vi "Shoot High Goal State Machine.vi"   [LabVIEW 2013]
uses:
  typedefs/DevRef Type.ctl
  typedefs/fg_typedef.ctl
  typedefs/State Machine/subStates.ctl
  typedefs/State Machine/singleUseSubstate.ctl
  <vilib>/Rock Robotics/WPI/Solenoid/WPI_SolenoidValue.ctl
  <vilib>/Rock Robotics/WPI/Solenoid/WPI_SolenoidGetEnum.vi
panel:
  # "A State Machine to Handle a High Goal Shot"
types:
  T1 = typedef "fg_typedef.ctl" = enum16{"Get", "Set"}
  T2 = typedef "DevRef Type.ctl" = enum16{"Shooter Solenoid", "Latch Solenoid", "Right Up Sensor", "Right Down Sensor", "Hold Sensor", "Arm Encoder"}
  T3 = typedef "subStates.ctl" = enum16{"null", "wait", "driver control", "auto", "manual override", "hold position", "rotate", "pickup", "pass", "recover pass", "load", "goto shoot", "shoot high goal", "shoot low goal", "cancel arm", "cancel shooter", "end", "test"}
  T4 = typedef "WPI_SolenoidValue.ctl" = enum16{"Off", "On", "Forward", "Reverse"}
  T5 = typedef "singleUseSubstate.ctl" = enum16{"null", "wait", "shift high", "shift low", "extend shooter", "retract shooter", "latch", "unlatch", "end"}
  T6 = typedef "WPI_DigitalInputDevRef.ctl" = cluster{"DevStatus":errorcluster, "DIO Channel":T7, "Digital Module":T8}
  T7 = typedef "FPGA_DIOChannel.ctl" = enum8{"DIO 1", "DIO 2", "DIO 3", "DIO 4", "DIO 5", "DIO 6", "DIO 7", "DIO 8", "DIO 9", "DIO 10", "DIO 11", "DIO 12", "DIO 13", "DIO 14", "Invalid"}
  T8 = typedef "FPGA_TypedefDigitalModule.ctl" = enum16{"Digital Module 1", "Digital Module 2"}
  T9 = typedef "WPI_SolenoidDevRef.ctl" = cluster{"DevStatus":errorcluster, "Solenoid Module":T10, "Forward Solenoid Channel":T11, "Reverse Solenoid Channel":T11}
  T10 = typedef "FPGA_TypedefSolenoidModule.ctl" = enum16{"Solenoid Module 1", "Solenoid Module 2"}
  T11 = typedef "WPI_SolenoidChannel.ctl" = enum8{"Solenoid 1", "Solenoid 2", "Solenoid 3", "Solenoid 4", "Solenoid 5", "Solenoid 6", "Solenoid 7", "Solenoid 8", "Invalid"}
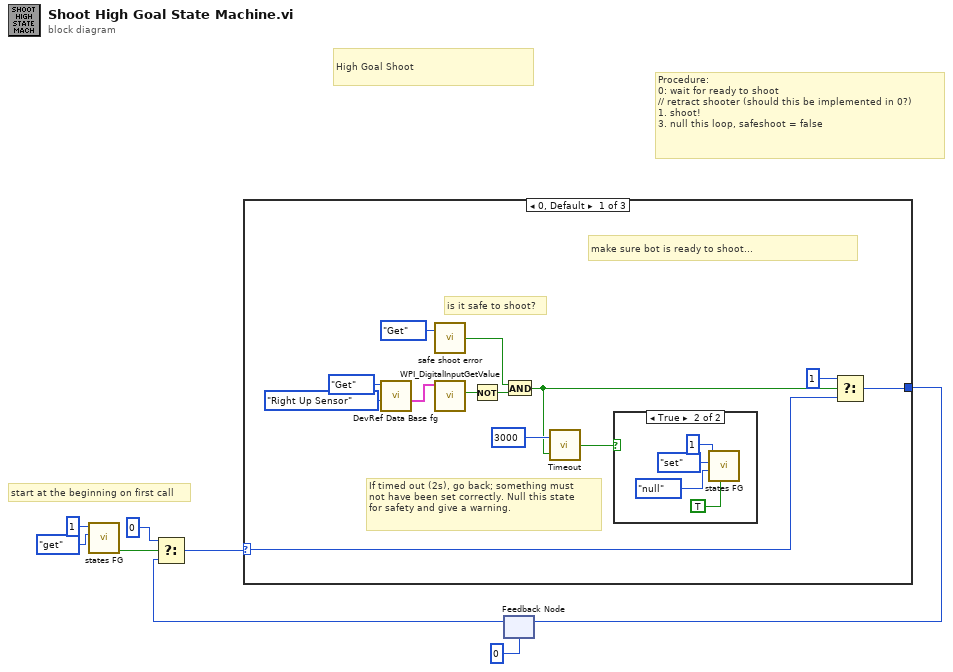
[diagram p0: block diagram]
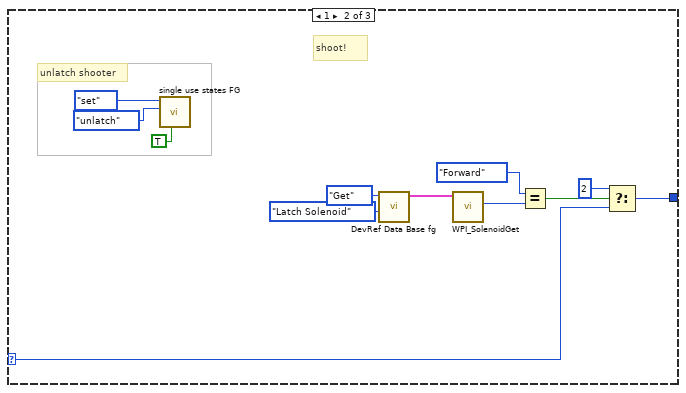
[diagram p3: hidden frame]
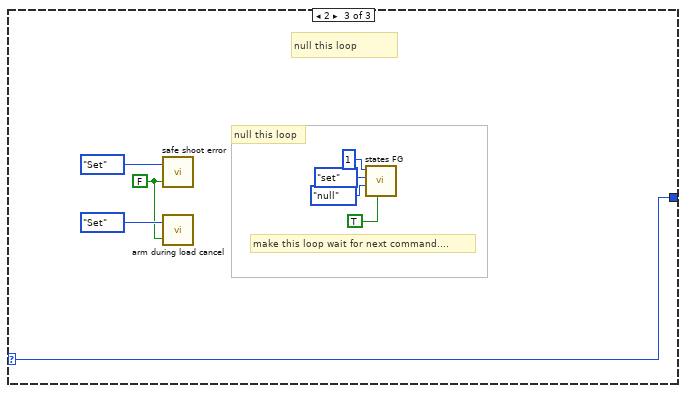
[diagram p4: hidden frame]
diagram:
  # "start at the beginning on first call"
  # "High Goal Shoot"
  # "Procedure:\n0: wait for ready to shoot\n// retract shooter (should this be implemented in 0?)\n1. shoot!\n3. null this loop, safeshoot = false"
  n1 = call "states FG.vi"("menu (get)"=enum16{"set", "get"}."get", "Loop ID"=1) -> ("first call?"=w1:bool)  [unwired: 6 in, 3 out]
  n2 = feedback #1(u8 0) -> (w4:u8)
  n3 = Select(t=u8 0, s=w1, f=w4) -> (s? t:f=w3:u8)
  n4 = case shown="0, Default" w3 {
    selector: w3 -> [w19 w30 w45]
    tunnel: [w20 w29 w45] -> w7
    frame 0, Default {
      # "If timed out (2s), go back; something must\nnot have been set correctly. Null this state\nfor safety and give a warning."
      # "is it safe to shoot?"
      # "make sure bot is ready to shoot..."
      n5 = call "DevRef Data Base fg.vi"("DevRef to Get"=DevRef_Type."Right Up Sensor", "Menu"=fg_typedef."Get") -> ("Selected Sensor"=w18:T6)  [unwired: 1 in, 8 out]
      n6 = call "safe shoot error.vi"("Menu"=fg_typedef."Get") -> ("Can Shoot Safely?"=w16:bool)  [unwired: 1 in]
      n7 = call <vilib>:"WPI_DigitalInputGetValue.vi"("DigitalInputDevRef"=w18) -> ("Value"=w21:bool)  [unwired: 8 in, 2 out]
      n8 = Not(x=w21) -> (.not. x?=w15:bool)
      n9 = And(x=w16, y=w15) -> (x .and. y?=w11:bool)
      n10 = call "Timeout.vi"("Done with Task?"=w11, "Timeout (ms)"=u32 3000) -> ("Timed Out?"=w12:bool)  [unwired: 1 in]
      n11 = case shown="True" w12 {
        frame False {
        }
        frame True {
          n12 = call "states FG.vi"("exit in"=TRUE, "subState in"=subStates."null", "menu (get)"=enum16{"set", "get"}."set", "Loop ID"=1) -> ()  [unwired: 4 in, 4 out]
        }
      }
      n13 = Select(t=u8 1, s=w11, f=w19) -> (s? t:f=w20:u8)
    }
    frame 1 {
      # "unlatch shooter"
      # "shoot!"
      n14 = call "single use states FG.vi"("exit in"=TRUE, "substate"=singleUseSubstate."unlatch", "menu (get)"=enum16{"set", "get"}."set") -> ()  [unwired: 5 in, 4 out]
      n15 = call "DevRef Data Base fg.vi"("DevRef to Get"=DevRef_Type."Latch Solenoid", "Menu"=fg_typedef."Get") -> ("Selected Solenoid"=w34:T9)  [unwired: 1 in, 8 out]
      n16 = call-poly <vilib>:"WPI_SolenoidGet.vi"("SolenoidDevRef"=w34) -> ("Value"=w33:T4)  [unwired: 8 in, 2 out]
      n17 = Equal?(x=WPI_SolenoidValue."Forward" ("Value"), y=w33) -> (x = y?=w31:bool)
      n18 = Select(t=u8 2, s=w31, f=w30) -> (s? t:f=w29:u8)
    }
    frame 2 {
      w38 = FALSE ("Can Shoot Safely?")
      # "null this loop"
      # "null this loop"
      # "make this loop wait for next command...."
      n19 = call "safe shoot error.vi"("Can Shoot Safely?"=w38, "Menu"=fg_typedef."Set") -> ()  [unwired: 1 out]
      n20 = call "arm during load cancel.vi"("Arm Canceled During Load?"=w38, "Mode"=enum16{"Get", "Set", "Teleop Set"}."Set") -> ()  [unwired: 1 out]
      n21 = call "states FG.vi"("exit in"=TRUE, "subState in"=subStates."null", "menu (get)"=enum16{"set", "get"}."set", "Loop ID"=1) -> ()  [unwired: 4 in, 4 out]
    }
  }
  n22 = feedback-in #1(w7) -> ()
